vi "encode_decode.vi"(1 "Enum":T1, 3 "Input string":string) -> (0 "encoded/decoded string":string)   [LabVIEW 2021]
uses:
  controls/encryption.ctl
panel:
  # "ägVVæ"
  # "ægVVæ"
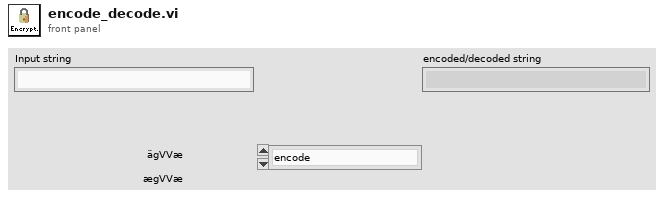
[diagram p1: front panel]
types:
  T1 = typedef "encryption.ctl" = enum16{"encode", "decode"}
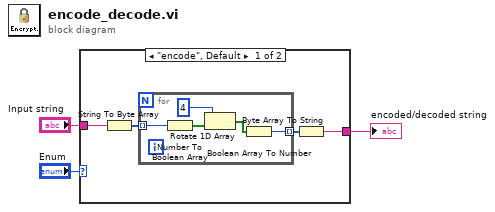
[diagram p0: block diagram]
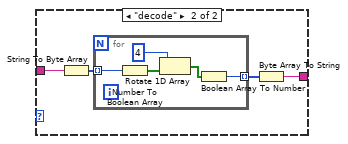
[diagram p2: hidden frame]
diagram:
  n1 = case shown="\"encode\", Default" "Enum" {
    tunnel: "Input string" -> [w7 w14]
    tunnel: [w4 w13] -> w2
    frame "encode", Default {
      n2 = String To Byte Array(string=w7) -> (unsigned byte array=w6:u8[])
      n3 = for {
        tunnel: w6 -> [w12] mode=indexing
        tunnel: [w8] -> w5 mode=indexing
        n4 = Number To Boolean Array(number=w12) -> (Boolean array=w11:bool[])
        n5 = Rotate 1D Array(1:w11, 2:4 ("n")) -> (0:w9:bool[])
        n6 = Boolean Array To Number(Boolean array=w9) -> (number=w8:u32)
      }
      n7 = Byte Array To String(unsigned byte array=w5) -> (string=w4:string)
    }
    frame "decode" {
      n8 = String To Byte Array(string=w14) -> (unsigned byte array=w15:u8[])
      n9 = for {
        tunnel: w15 -> [w21] mode=indexing
        tunnel: [w17] -> w16 mode=indexing
        n10 = Number To Boolean Array(number=w21) -> (Boolean array=w20:bool[])
        n11 = Rotate 1D Array(1:w20, 2:4 ("n")) -> (0:w18:bool[])
        n12 = Boolean Array To Number(Boolean array=w18) -> (number=w17:u32)
      }
      n13 = Byte Array To String(unsigned byte array=w16) -> (string=w13:string)
    }
  }
  "encoded/decoded string" <- w2
